vi "Remove Node.vi"(8 "error in (no error)":errorcluster, 10 "Node Path (parent, child)":string[](array[string]), 11 "Tree Map Handle In":T1) -> (0 "error out":errorcluster, 2 "Node Removed?":bool, 3 "Tree Map Handle Out":T1)   [LabVIEW 2020, in "Blue Tree Map OpenSource.lvlib"]
doc: "This will remove the specified node path if it exists.\nAll children will also be removed."
uses:
  Blue Tree Map OpenSource.lvlib
  Typedefs/Tree Map Handle.ctl
  Typedefs/Tree Map.ctl
  Typedefs/Tree Map Data.ctl
  Typedefs/Tree Node Data.ctl
  Typedefs/Attribute Map.ctl
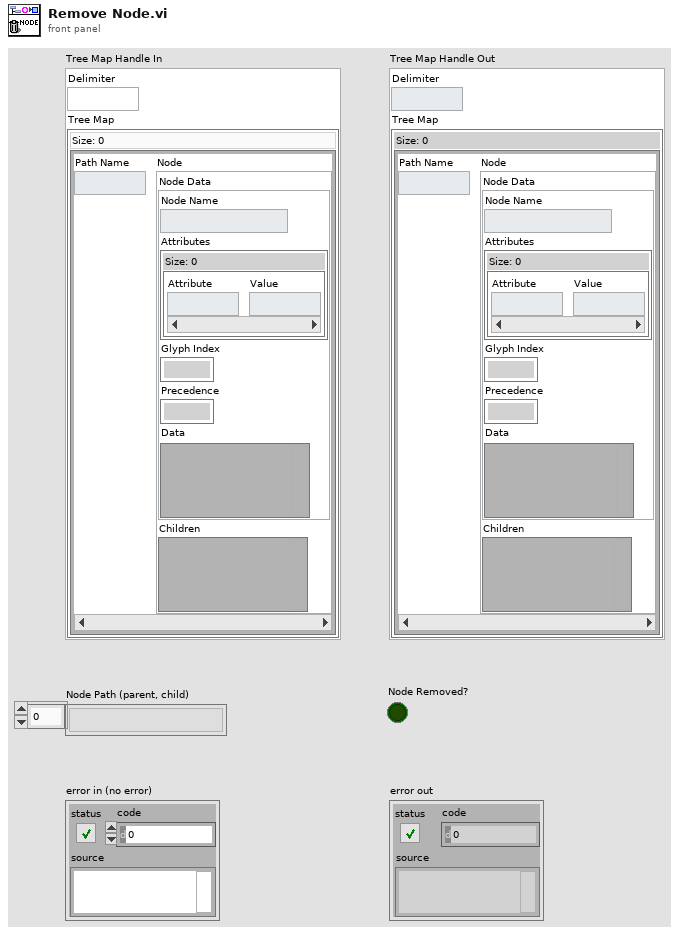
[diagram p1: front panel]
types:
  T1 = typedef "Blue Tree Map OpenSource.lvlib/Tree Map Handle.ctl" = cluster{"Delimiter":string, "Tree Map":T2}
  T2 = typedef "Blue Tree Map OpenSource.lvlib/Tree Map.ctl" = map{string, T3}
  T3 = typedef "Blue Tree Map OpenSource.lvlib/Tree Map Data.ctl" = cluster{"Node Data":T4, "Children":variant}
  T4 = typedef "Blue Tree Map OpenSource.lvlib/Tree Node Data.ctl" = cluster{"Node Name":string, "Attributes":T5, "Glyph Index":i32, "Precedence":i32, "Data":variant}
  T5 = typedef "Blue Tree Map OpenSource.lvlib/Attribute Map.ctl" = map{string, string}
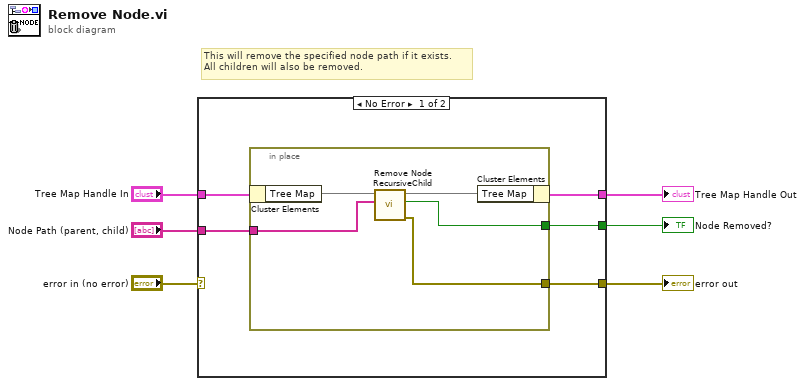
[diagram p0: block diagram]
diagram:
  # "This will remove the specified node path if it exists.\nAll children will also be removed."
  n1 = case shown="No Error" "error in (no error)" {
    selector: "error in (no error)" -> [_ w18]
    tunnel: "Node Path (parent, child)" -> [w11 _]
    tunnel: [w10 w18] -> w5
    tunnel: [w9 _] -> w4
    tunnel: "Tree Map Handle In" -> [w8 w17]
    tunnel: [w7 w17] -> w2
    frame No Error {
      n2 = in-place {
        in-place-border: w11 -> [w14]
        in-place-border: [w13] -> w10
        in-place-border: [w12] -> w9
        n3 = in-place-cluster #1(w8) -> ("Tree Map"=w16:T2)
        n4 = call "Remove Node RecursiveChild.vi"("New Node Path (parent, child)"=w14, "Tree Map In"=w16) -> ("error out"=w13:errorcluster, "Node removed?"=w12:bool, "Tree Map Out"=w15:T2)  [unwired: 7 in]
        n5 = in-place-cluster #1("Tree Map"=w15) -> (w7:T1)
      }
    }
    frame Error {
    }
  }
  "error out" <- w5
  "Node Removed?" <- w4
  "Tree Map Handle Out" <- w2
